vi "arduino_commands_2.vi"(1 "Número de motor":string, 2 "Argumento":string, 3 "Directorio scripts ArduinoStepper.py":path=path "C:/Users/franjas/Documents/rutinas-calibracion-slm", 4 "wait until completion? (T)":bool=TRUE, 5 "Set speed":bool) -> ()   [LabVIEW 2013]
panel:
  in  "Comando":string
  out "Comando que está siendo enviado a python":string
  out "standard output":string
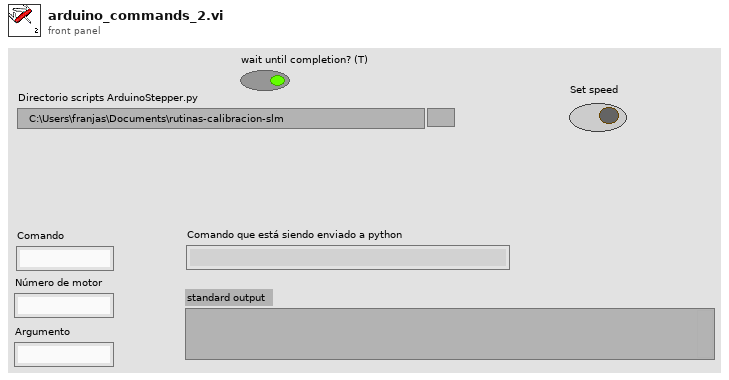
[diagram p1: front panel]
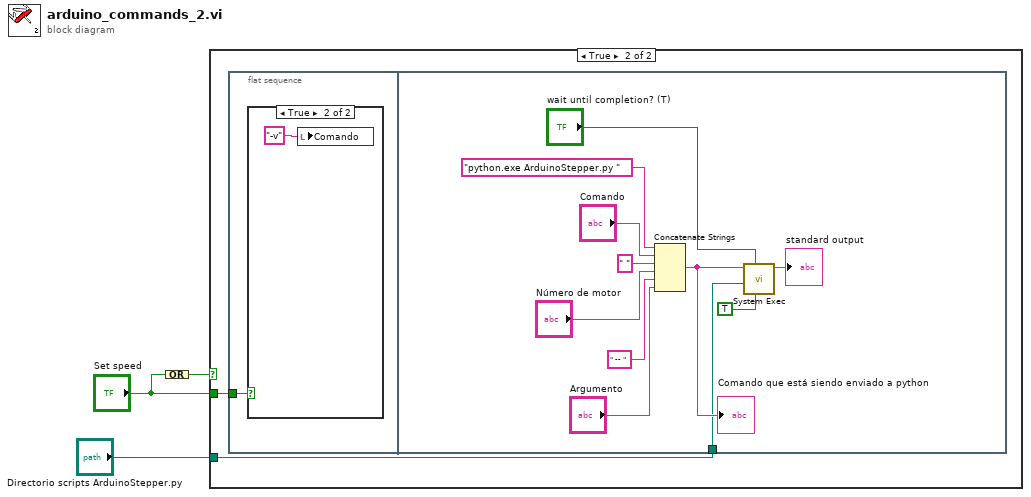
[diagram p0: block diagram]
diagram:
  n1 = Compound Arithmetic op=OR("Set speed") -> (w3:bool)
  n2 = case shown="True" w3 {
    tunnel: "Set speed" -> [_ w5]
    tunnel: "Directorio scripts ArduinoStepper.py" -> [_ w4]
    frame False {
    }
    frame True {
      n3 = flat-sequence {
        tunnel: w5 -> [w6]
        tunnel: w4 -> [w8]
        frame #0 {
          n4 = case shown="True" w6 {
            frame False {
            }
            frame True {
              n5 = local write "Comando"("-v" ("Comando")) -> ()
            }
          }
        }
        frame #1 {
          n6 = Concatenate Strings("python.exe ArduinoStepper.py ", "Comando", " " ("string"), "Número de motor", " -- ", "Argumento") -> (w12:string)
          "Comando que está siendo enviado a python" <- w12
          n7 = call <vilib>:"System Exec.vi"("run minimized? (F)"=TRUE, "wait until completion? (T)"="wait until completion? (T)", "working directory"=w8, "command line"=w12) -> ("standard output"=→"standard output":string)  [unwired: 4 in, 3 out]
        }
      }
    }
  }
